vi "PWMFeedDog.vi"(8 "ErrorIn(no error)":errorcluster, 11 "FPGA VI引用输入":refnum<k20>) -> (0 "ErrorOut":errorcluster, 3 "FPGA VI引用输出":refnum<k20>)   [LabVIEW 2015]
uses:
  <vilib>/Utility/error.llb/Error Cluster From Error Code.vi
  <vilib>/rvi/errors/niLvFpgaAdjustHostInterfaceError.vi
  <vilib>/rvi/interface/nirviReadWriteControl/nirviReadWriteControl.xnode
  NiFpgaLv.dll
  <vilib>/rvi/interface/Simulation/niFpgaSimulationCallBeginRW.vi
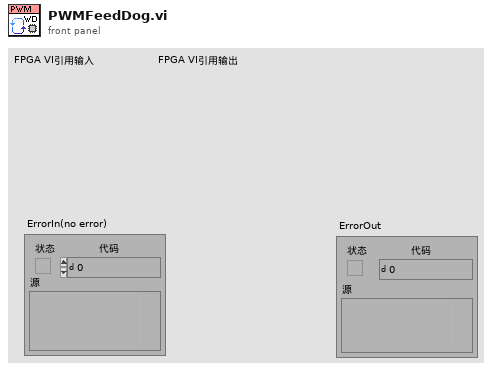
[diagram p1: front panel]
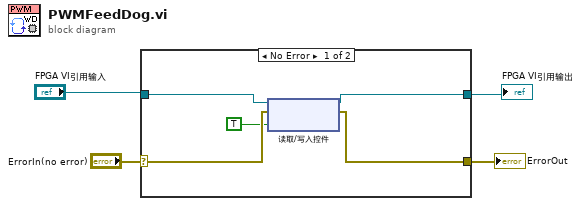
[diagram p0: block diagram]
diagram:
  n1 = case shown="No Error" "ErrorIn(no error)" {
    selector: "ErrorIn(no error)" -> [w8 w10]
    tunnel: "FPGA VI引用输入" -> [w9 w11]
    tunnel: [w6 w11] -> w1
    tunnel: [w5 w10] -> w3
    frame No Error {
      n2 = xnode "读取/写入控件"("FPGA VI Reference In"=w9, "error in"=w8, "FeedDog"=TRUE) -> ("FPGA VI Reference Out"=w6:refnum<k20>, "error out"=w5:errorcluster)
    }
    frame Error {
    }
  }
  "ErrorOut" <- w3
  "FPGA VI引用输出" <- w1
